vi "RUSHShoot.vi"(1 "In Cluster":T3={"ShootTrackEnable"=FALSE, "ShootStartWheels"=FALSE, "ShootIndexerEnable"=FALSE, "ShootCase"=0.0, "ShootPOTElev"=0.0, "ShootManualElev"=0.0, "Wheel Spd F"=0.0, "Deadband"=0.0, "ShootConstElev"={"1"=0.0, "2"=0.0, "3"=0.0, "4"=0.0, "Ground"=0.0}, "ShootRollerSpd"=0.0, "ShootFlipperPE"=FALSE, "Wheel Spd B"=0.0, "ShootConstFlipper"={"Down 1"=0.2, "Up 1"=0.8, "Up 2"=0.8, "Down 2"=0.2}, "Y Coord"=0.0, "ShootConstIndexer"={"Pushed"=0.2, "Normal"=0.8}}) -> (0 "Out Cluster":T2)   [LabVIEW 2012]
uses:
  <vilib>/Rock Robotics/WPI/Relay/WPI_RelayValue.ctl
panel:
  in  "Highest POT pos":dbl=4.2
  in  "Lowest POT pos":dbl=2.1
  in  "ShootPOTToPowConst":dbl=1.0
  in  "Vision Speed Const":dbl=0.75
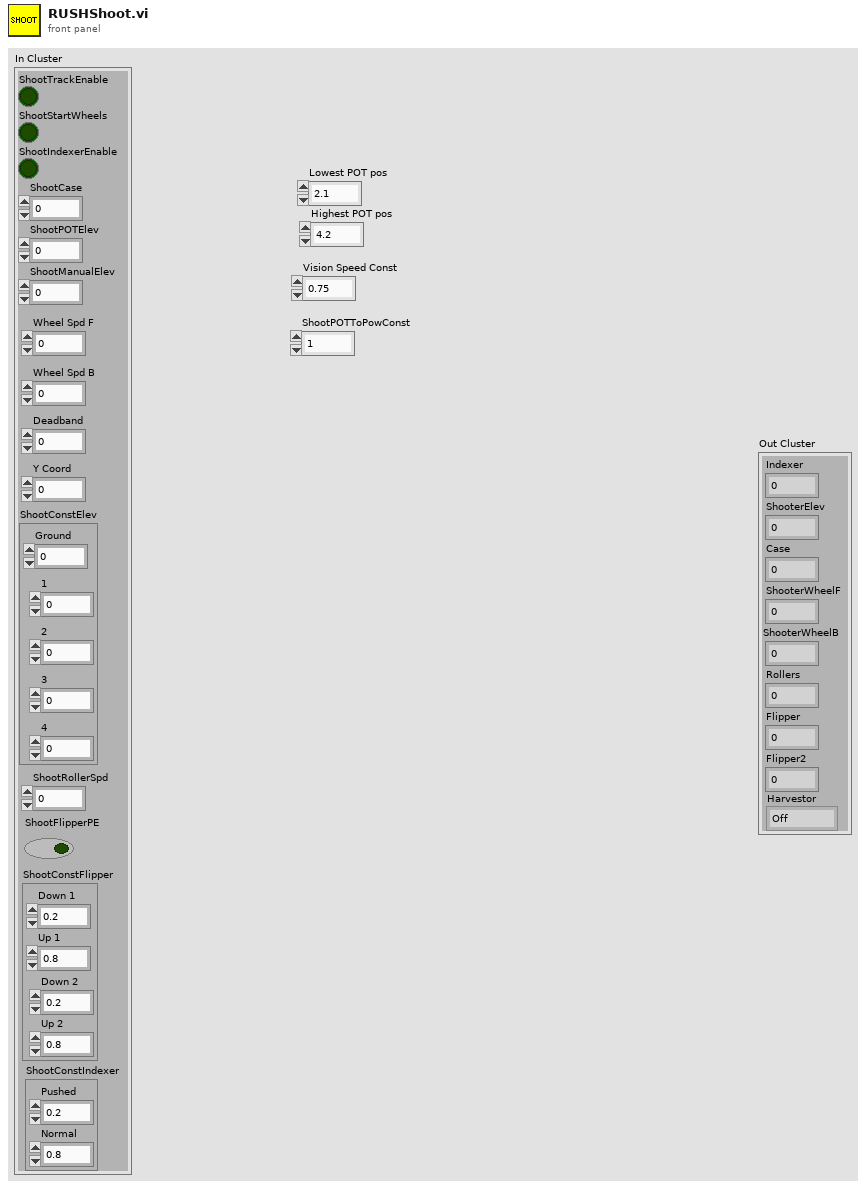
[diagram p1: front panel]
types:
  T1 = typedef "WPI_RelayValue.ctl" = enum16{"Off", "On", "Forward", "Reverse"}
  T2 = cluster{"Indexer":dbl, "ShooterElev":dbl, "Case":dbl, "ShooterWheelF":dbl, "ShooterWheelB":dbl, "Rollers":dbl, "Flipper":dbl, "Flipper2":dbl, "Harvestor":T1}
  T3 = cluster{"ShootTrackEnable":bool, "ShootStartWheels":bool, "ShootIndexerEnable":bool, "ShootCase":dbl, "ShootPOTElev":dbl, "ShootManualElev":dbl, "Wheel Spd F":dbl, "Deadband":dbl, "ShootConstElev":cluster{"1":dbl, "2":dbl, "3":dbl, "4":dbl, "Ground":dbl}, "ShootRollerSpd":dbl, "ShootFlipperPE":bool, "Wheel Spd B":dbl, "ShootConstFlipper":cluster{"Down 1":dbl, "Up 1":dbl, "Up 2":dbl, "Down 2":dbl}, "Y Coord":dbl, "ShootConstIndexer":cluster{"Pushed":dbl, "Normal":dbl}}
  T4 = cluster{"1":dbl, "2":dbl, "3":dbl, "4":dbl, "Ground":dbl}
  T5 = cluster{"Down 1":dbl, "Up 1":dbl, "Up 2":dbl, "Down 2":dbl}
  T6 = cluster{"f":dbl, "y":dbl, "f":dbl, "f":dbl, "f":dbl, "f":dbl, "Down 1":dbl, "Down 2":dbl, "Harvestor":T1}
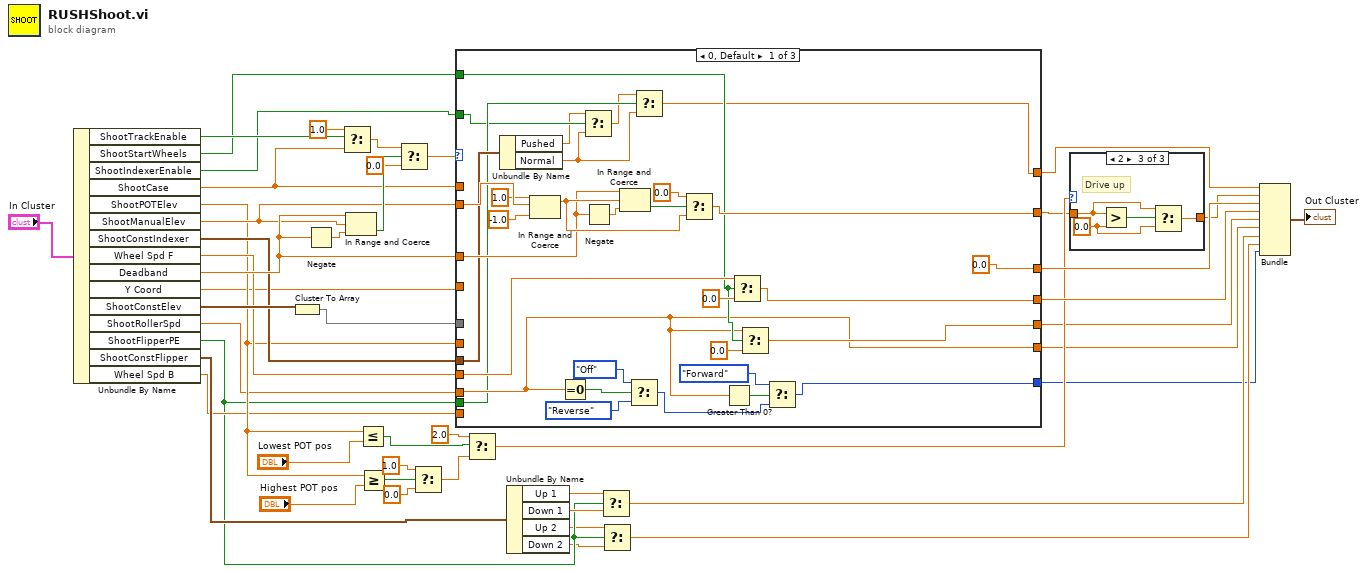
[diagram p0: block diagram]
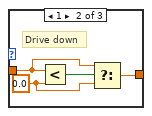
[diagram p3: hidden frame]
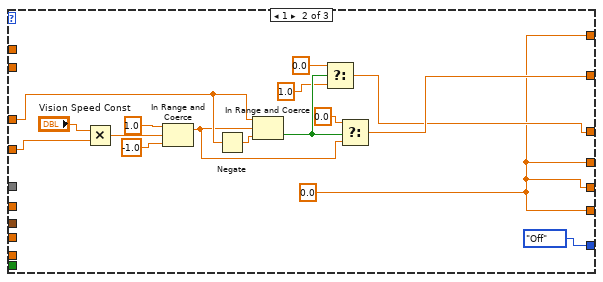
[diagram p4: hidden frame]
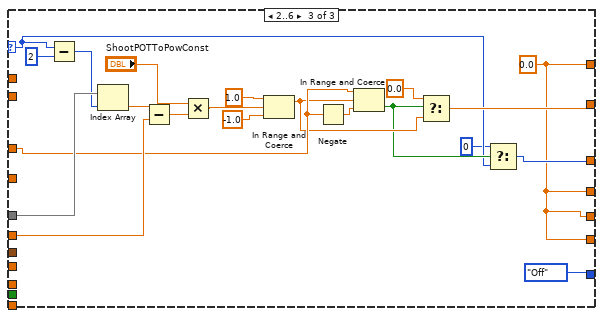
[diagram p5: hidden frame]
diagram:
  n1 = Unbundle By Name("In Cluster") -> ("ShootTrackEnable"=w46:bool, "ShootStartWheels"=w37:bool, "ShootIndexerEnable"=w36:bool, "ShootCase"=w38:dbl, "ShootPOTElev"=w26:dbl, "ShootManualElev"=w35:dbl, "ShootConstIndexer"=w29:cluster{"Pushed":dbl, "Normal":dbl}, "Wheel Spd F"=w28:dbl, "Deadband"=w39:dbl, "Y Coord"=w1:dbl, "ShootConstElev"=w34:T4, "ShootRollerSpd"=w15:dbl, "ShootFlipperPE"=w7:bool, "ShootConstFlipper"=w13:T5, "Wheel Spd B"=w11:dbl)
  n2 = Cluster To Array(cluster=w34) -> (array=w33:dbl[])
  n3 = Negate(x=w39) -> (-x=w43:dbl)
  n4 = Select(t=1.0, s=w46, f=w38) -> (s? t:f=w44:dbl)
  n5 = In Range and Coerce(upper limit=w39, x=w35, lower limit=w43) -> (In Range?=w42:bool)  [unwired: 1 out]
  n6 = Less Or Equal?(x=w26, y="Lowest POT pos") -> (x <= y?=w20:bool)
  n7 = Greater Or Equal?(x=w26, y="Highest POT pos") -> (x >= y?=w24:bool)
  n8 = Select(t=w44, s=w42, f=0.0) -> (s? t:f=w40:dbl)
  n9 = Select(t=1.0, s=w24, f=0.0) -> (s? t:f=w21:dbl)
  n10 = case shown="0, Default" w40 {
    selector: w40 -> [_ _ w99]
    tunnel: w1 -> [_ w93 _]
    tunnel: w39 -> [w66 w88 w104]
    tunnel: [0.0 ("upper limit") w82 w97] -> w31
    tunnel: w38 -> [_ _ _]
    tunnel: [w72 w83 w101] -> w17
    tunnel: [w70 w80 w96] -> w30
    tunnel: [w48 w80 w96] -> w32
    tunnel: w37 -> [w64 _ _]
    tunnel: w36 -> [w52 _ _]
    tunnel: w35 -> [w76 _ _]
    tunnel: w33 -> [_ _ w114]
    tunnel: w26 -> [_ _ w111]
    tunnel: w29 -> [w54 _ _]
    tunnel: w28 -> [w67 _ _]
    tunnel: w15 -> [w55 _ _]
    tunnel: [w55 w80 w96] -> w9
    tunnel: w7 -> [w53 _ _]
    tunnel: w11 -> [_ _ _]
    tunnel: [w63 w80 w96] -> w8
    tunnel: [w56 WPI_RelayValue."Off" ("Harvestor") WPI_RelayValue."Off" ("Harvestor")] -> w3
    frame 0, Default {
      n11 = Unbundle By Name(w54) -> ("Pushed"=w51:dbl, "Normal"=w49:dbl)
      n12 = In Range and Coerce(upper limit=1.0, x=w76, lower limit=-1.0 ("upper limit")) -> (coerced(x)=w73:dbl)  [unwired: 1 out]
      n13 = Equal To 0?(x=w55) -> (x = 0?=w60:bool)
      n14 = Select(t=w51, s=w52, f=w49) -> (s? t:f=w50:dbl)
      n15 = Negate(x=w66) -> (-x=w77:dbl)
      n16 = In Range and Coerce(upper limit=w66, x=w73, lower limit=w77) -> (In Range?=w75:bool)  [unwired: 1 out]
      n17 = Select(t=WPI_RelayValue."Off" ("Harvestor"), s=w60, f=WPI_RelayValue."Reverse" ("Harvestor")) -> (s? t:f=w57:T1)
      n18 = Select(t=w50, s=w53, f=w49) -> (s? t:f=w48:dbl)
      n19 = Select(t=0.0, s=w75, f=w73) -> (s? t:f=w72:dbl)
      n20 = Greater Than 0?(x=w55) -> (x > 0?=w62:bool)
      n21 = Select(t=w67, s=w64, f=0.0 ("t")) -> (s? t:f=w70:dbl)
      n22 = Select(t=w55, s=w64, f=0.0 ("t")) -> (s? t:f=w63:dbl)
      n23 = Select(t=WPI_RelayValue."Forward" ("Harvestor"), s=w62, f=w57) -> (s? t:f=w56:T1)
    }
    frame 1 {
      w80 = 0.0
      n24 = Multiply(x="Vision Speed Const", y=w93) -> (x*y=w92:dbl)
      n25 = In Range and Coerce(upper limit=1.0, x=w92, lower limit=-1.0 ("upper limit")) -> (coerced(x)=w86:dbl)  [unwired: 1 out]
      n26 = Negate(x=w88) -> (-x=w89:dbl)
      n27 = In Range and Coerce(upper limit=w88, x=w86, lower limit=w89) -> (In Range?=w85:bool)  [unwired: 1 out]
      n28 = Select(t=0.0, s=w85, f=1.0) -> (s? t:f=w82:dbl)
      n29 = Select(t=0.0, s=w85, f=w86) -> (s? t:f=w83:dbl)
    }
    frame 2..6 {
      w96 = 0.0 ("f")
      n30 = Subtract(x=w99, y=2) -> (x-y=w113:i32)
      n31 = Index Array(array=w114, index=w113) -> (element=w112:dbl)
      n32 = Subtract(x=w112, y=w111) -> (x-y=w110:dbl)
      n33 = Multiply(x="ShootPOTToPowConst", y=w110) -> (x*y=w105:dbl)
      n34 = In Range and Coerce(upper limit=1.0, x=w105, lower limit=-1.0 ("upper limit")) -> (coerced(x)=w102:dbl)  [unwired: 1 out]
      n35 = Negate(x=w104) -> (-x=w106:dbl)
      n36 = In Range and Coerce(upper limit=w104, x=w102, lower limit=w106) -> (In Range?=w100:bool)  [unwired: 1 out]
      n37 = Select(t=0.0, s=w100, f=w102) -> (s? t:f=w101:dbl)
      n38 = Select(t=0, s=w100, f=w99) -> (s? t:f=w97:i32)
    }
  }
  n39 = Select(t=2.0, s=w20, f=w21) -> (s? t:f=w18:dbl)
  n40 = Unbundle By Name(w13) -> ("Up 1"=w12:dbl, "Down 1"=w14:dbl, "Up 2"=w6:dbl, "Down 2"=w5:dbl)
  n41 = Select(t=w12, s=w7, f=w14) -> (s? t:f=w10:dbl)
  n42 = Select(t=w6, s=w7, f=w5) -> (s? t:f=w4:dbl)
  n43 = case shown="2" w18 {
    tunnel: w17 -> [w116 w118 w122]
    tunnel: [w116 w117 w121] -> w16
    frame 0, Default {
      # "All good"
    }
    frame 1 {
      w119 = 0.0 ("y")
      # "Drive down"
      n44 = Less?(x=w118, y=w119) -> (x < y?=w120:bool)
      n45 = Select(t=w118, s=w120, f=w119) -> (s? t:f=w117:dbl)
    }
    frame 2 {
      w123 = 0.0 ("y")
      # "Drive up"
      n46 = Greater?(x=w122, y=w123) -> (0:w124:bool)
      n47 = Select(t=w122, s=w124, f=w123) -> (s? t:f=w121:dbl)
    }
  }
  n48 = Bundle("f"=w32, "y"=w16, "f"=w31, "f"=w30, "f"=w8, "f"=w9, "Down 1"=w10, "Down 2"=w4, "Harvestor"=w3) -> (→"Out Cluster":T6)  [unwired: 1 in]
